vi "PalmSense Action-Status Switch.vi"(8 "error in (no error)":errorcluster, 10 "Message Data":variant, 11 "Data Cluster in":T1) -> (0 "error out":errorcluster, 3 "Data Cluster out":T1)   [LabVIEW 2020, in "PalmSens.lvlib"]
uses:
  PalmSens.lvlib
  support/HW Message Cluster.ctl
  support/Message Queue/Message Queue.lvlib
  support/Message Queue/Message Cluster.ctl
  PalmSense Hardware Configuration.ctl
  Program Files (x86)/National Instruments/LabVIEW 2023/instr.lib/PalmSens SDK for LabVIEW 5.10/PalmSens/PalmSens.lvclass
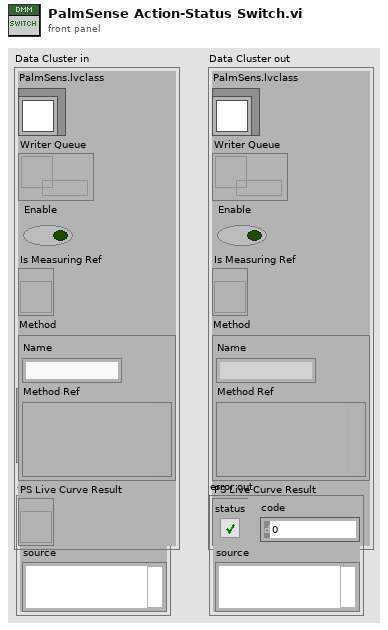
[diagram p1: front panel]
types:
  T1 = typedef "PalmSens.lvlib/PalmSense Hardware Configuration.ctl" = cluster{"PalmSens.lvclass":refnum<class "PalmSens.lvclass">, "Writer Queue":refnum<queue>, "Enable":bool, "Is Measuring Ref":refnum<vi>, "Method":cluster{"Name":string, "Method Ref":variant}, "PS Live Curve Result":refnum<vi>}
  T2 = typedef "Message Queue.lvlib/HW Message Cluster.ctl" = cluster{"Writer Queue":refnum<queue>, "Writer Data":T3}
  T3 = typedef "Message Queue.lvlib/Message Cluster.ctl" = cluster{"Message":string, "Message Data":variant}
  T4 = cluster{"Set/Check (F:Set)":bool, "Open/Close (F:Close)":bool, "Close Exclusive (F:Normal)":bool, "Channel List(empty)":string}
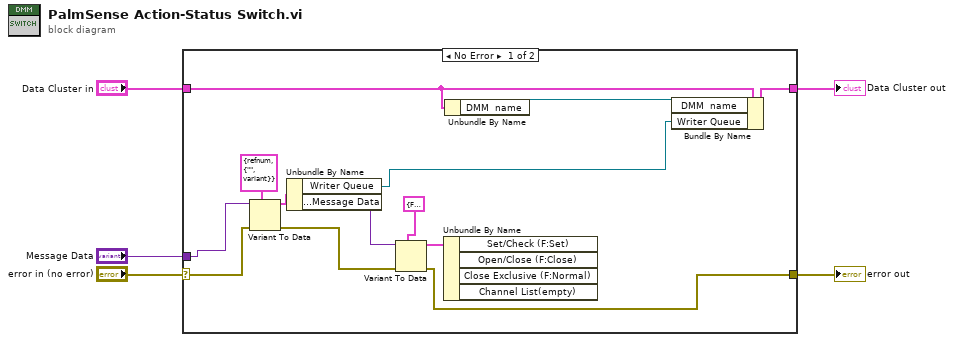
[diagram p0: block diagram]
diagram:
  n1 = case shown="No Error" "error in (no error)" {
    selector: "error in (no error)" -> [w10 w19]
    tunnel: "Message Data" -> [w8 _]
    tunnel: [w16 w20] -> w4
    tunnel: "Data Cluster in" -> [w15 w20]
    tunnel: [w18 w19] -> w2
    frame No Error {
      n2 = Variant To Data(error in=w10, type=T2 {"Writer Queue"=refnum, "Writer Data"={"Message"="", "Message Data"=variant}}, Variant=w8) -> (data=w11:T2, error out=w9:errorcluster)
      n3 = Unbundle By Name(w11) -> ("Writer Queue"=w6:refnum<queue>, "Writer Data.Message Data"=w7:variant)
      n4 = Variant To Data(error in=w9, type=T4 {"Set/Check (F:Set)"=FALSE, "Open/Close (F:Close)"=FALSE, "Close Exclusive (F:Normal)"=FALSE, "Channel List(empty)"=""}, Variant=w7) -> (data=w13:T4, error out=w18:errorcluster)
      n5 = Unbundle By Name(w13) -> ()  [unwired: 4 out]
      n6 = Unbundle By Name(w15) -> ("DMM  name"=w17:refnum<visa-resource-name>)
      n7 = Bundle By Name(cluster=w15, "DMM  name"=w17, "Writer Queue"=w6) -> (w16:T1)
    }
    frame Error {
    }
  }
  "Data Cluster out" <- w4
  "error out" <- w2
